vi "WaitPassTactic_v2_Init.vi"(0 "object in":refnum<class "WaitPassTactic_v2.lvclass">, 5 "error in (no error)":errorcluster) -> (14 "object out":refnum<class "WaitPassTactic_v2.lvclass">, 19 "error out":errorcluster)   [LabVIEW 2023, in "WaitPassTactic_v2.lvclass"]
uses:
  WaitPassTactic_v2.lvclass
  C:/Users/ebert/Documents/codes/SSL/repo/SSL_AI/NewSTP/NewTactics/Tactic_v2_class/Tactic_v2.lvclass
  NewSTP/NewSkills/HaltSkill_v2_class/HaltSkill_v2.lvclass
  C:/Users/ebert/Documents/codes/SSL/repo/SSL_AI/NewSTP/NewSkills/Skill_v2_class/Skill_v2.lvclass
  NewSTP/NewTactics/Tactic_v2_class/Tactic_v2.lvclass
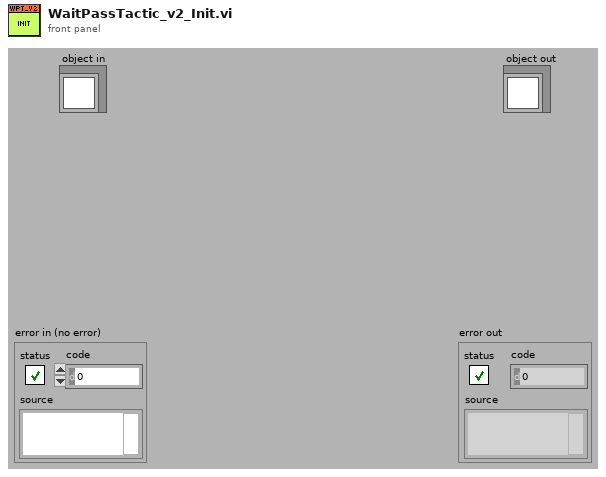
[diagram p1: front panel]
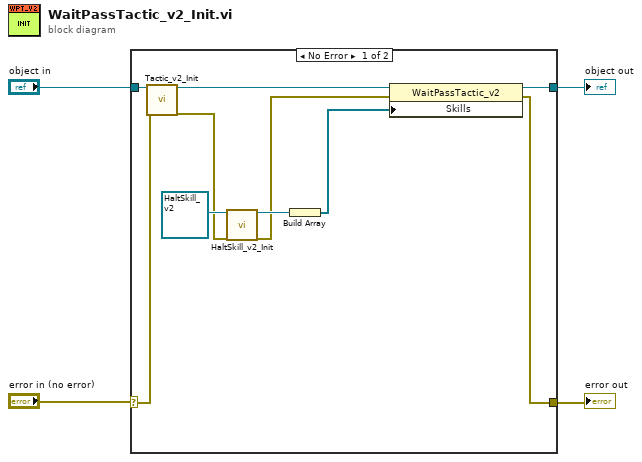
[diagram p0: block diagram]
diagram:
  n1 = case shown="No Error" "error in (no error)" {
    selector: "error in (no error)" -> [w13 w15]
    tunnel: "object in" -> [w14 w16]
    tunnel: [w6 w16] -> w3
    tunnel: [w5 w15] -> w1
    frame No Error {
      n2 = call "Tactic_v2_Init.vi"("object in"=w14, "error in (no error)"=w13) -> ("object out"=w8:refnum<class "WaitPassTactic_v2.lvclass">, "error out"=w11:errorcluster)  [unwired: 16 in]
      n3 = call "HaltSkill_v2_Init.vi"("object in"=refnum<class "HaltSkill_v2.lvclass"> refnum ("HaltSkill_v2"), "error in (no error)"=w11) -> ("object out"=w10:refnum<class "HaltSkill_v2.lvclass">, "error out"=w9:errorcluster)  [unwired: 16 in]
      n4 = Build Array(w10) -> (w7:refnum<class "HaltSkill_v2.lvclass">[])
      n5 = property class="WaitPassTactic_v2"(reference=w8, error in=w9, "Skills"=w7) -> (reference out=w6:refnum<class "WaitPassTactic_v2.lvclass">, error out=w5:errorcluster)
    }
    frame Error {
    }
  }
  "object out" <- w3
  "error out" <- w1
